vi "GenerateSineSignal.vi"() -> (3 "Sine with Poisson Noise":dynamicdata(graph))   [LabVIEW 2010]
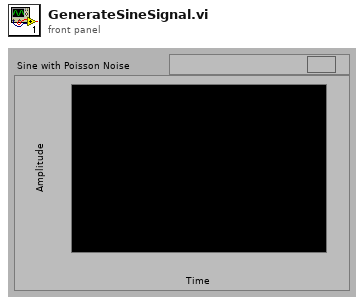
[diagram p1: front panel]
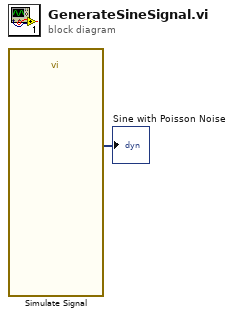
[diagram p0: block diagram]
diagram:
  n1 = call "Simulate Signal"() -> ("Sine with Poisson Noise"=→"Sine with Poisson Noise":dynamicdata)  [unwired: 14 in, 1 out]
